vi "BT_Reader.vi"() -> ()   [LabVIEW 2016]
doc: "Demonstrates how to open a connection to a specified Bluetooth server and channel, read the data being sent to the channel, and display the data on a chart. This VI is designed to stop if the Bluetooth connection is terminated."
panel:
  out "Packet Count":i32
  out "String":string
  out "Channel":u16
  in  "Device Name":string="HAILO"
  in  "Stop":bool
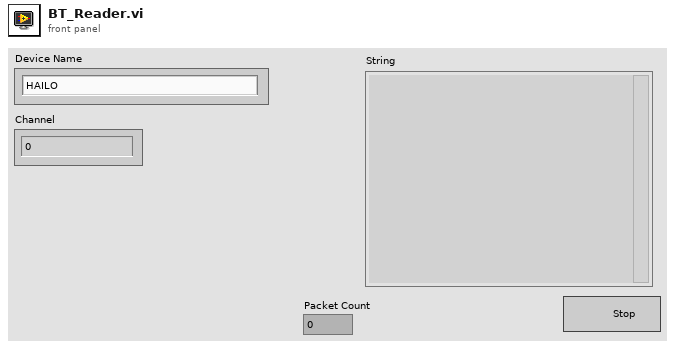
[diagram p1: front panel]
types:
  T1 = cluster{"channel":u16, "uuid":string, "service name":string, "service description":string}[]
  T2 = cluster{"channel":u16, "uuid":string, "service name":string, "service description":string}
  T3 = enum16{"Standard", "Buffered", "CRLF", "Immediate"}
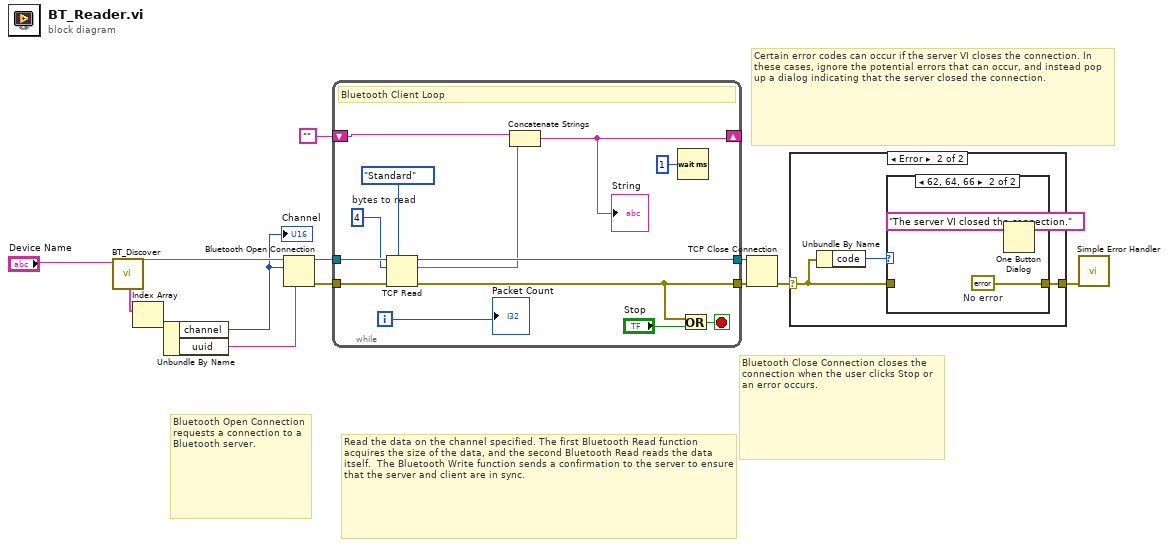
[diagram p0: block diagram]
diagram:
  # "Certain error codes can occur if the server VI closes the connection. In these cases, ignore the potential errors that can occur, and instead pop up a dialog indicating that the server closed the connection."
  # "Bluetooth Close Connection closes the connection when the user clicks Stop or an error occurs."
  # "Read the data on the channel specified. The first Bluetooth Read function acquires the size of the data, and the second Bluetooth Read reads the data itself.  The Bluetooth Write function sends a confirmation to the server to ensure that the server and client are in sync."
  # "Bluetooth Open Connection requests a connection to a Bluetooth server."
  n1 = call "BT_Discover.vi"("Device Name"="Device Name") -> ("Device Address"=w6:string, "service list"=w4:T1)  [unwired: 6 in, 3 out]
  n2 = Index Array(array=w4) -> (element=w3:T2)  [unwired: 1 in]
  n3 = Unbundle By Name(w3) -> ("channel"=w2:u16, "uuid"=w1:string)
  "Channel" <- w2
  n4 = Bluetooth Open Connection(6:w1, 10:w2, 11:w6) -> (0:w12:errorcluster, 3:w13:refnum<k31>)  [unwired: 2 in]
  n5 = while {
    tunnel: w12 -> [w25]
    tunnel: w13 -> [w26]
    tunnel: [w16] -> w9
    tunnel: [w20] -> w8
    shift-right: [w19] -> _
    shift-left: "" -> [w18]
    i -> [w14]
    stop <- w23 stop-if-true
    w21 = 4  # bytes to read
    # "Bluetooth Client Loop"
    n6 = TCP Read(connection ID=w26, bytes to read=w21, error in (no error)=w25, 7:T3."Standard" ("mode (standard)")) -> (connection ID out=w20:refnum<k31>, data out=w17:string, error out=w16:errorcluster)  [unwired: 1 in]
    n7 = Concatenate Strings(w18, w17) -> (w19:string)
    "String" <- w19
    n8 = Wait (ms)(milliseconds to wait=u32 1) -> ()  [unwired: 1 out]
    n9 = Or(x=w16, y="Stop") -> (x .or. y?=w23:bool)
    "Packet Count" <- w14
  }
  n10 = TCP Close Connection(connection ID=w8, error in (no error)=w9) -> (error out=w11:errorcluster)  [unwired: 1 in, 1 out]
  n11 = case shown="Error" w11 {
    selector: w11 -> [w27 w29]
    tunnel: [w27 w28] -> w10
    frame No Error {
    }
    frame Error {
      n12 = Unbundle By Name(w29) -> ("code"=w30:i32)
      n13 = case shown="62, 64, 66" w30 {
        tunnel: w29 -> [w31 _]
        tunnel: [w31 w33] -> w28
        frame Default {
        }
        frame 62, 64, 66 {
          w33 = errorcluster {"status"=FALSE, "code"=0, "source"=""}  # No error
          n14 = One Button Dialog(message="The server VI closed the connection." ("Server Closed")) -> ()  [unwired: 1 in, 1 out]
        }
      }
    }
  }
  n15 = call <vilib>:"Simple Error Handler.vi"("error in (no error)"=w10) -> ()  [unwired: 4 in, 5 out]
